vi "Setup.vi"(8 "error in":errorcluster, 11 "LUnit Test Commands In":refnum<class "Test Commands.lvclass">) -> (0 "error out":errorcluster, 3 "LUnit Test Commands Out":refnum<class "Test Commands.lvclass">)   [LabVIEW 2019, in "Test Commands.lvclass"]
doc: "Setup method called by the testing framework to set up test fixture before each test method is called."
uses:
  Test Commands.lvclass
  Test Commands.lvclass/Test Commands.ctl
  <vilib>/Astemes/LUnit/Test Case.lvclass
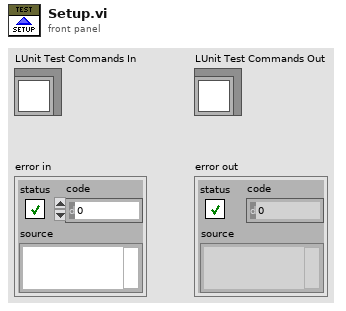
[diagram p1: front panel]
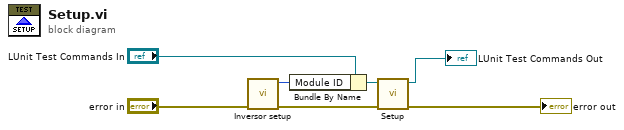
[diagram p0: block diagram]
diagram:
  n1 = call "Inversor setup.vi"("error in (no error)"="error in") -> ("error out"=w5:errorcluster, "Module ID"=w1:i32)  [unwired: 9 in]
  n2 = Bundle By Name(cluster="LUnit Test Commands In", "Module ID"=w1) -> (w2:refnum<class "Test Commands.lvclass">)
  n3 = call-parent "Setup.vi"("error in (no error)"=w5, "LUnit Test Case In"=w2) -> ("error out"=→"error out":errorcluster, "LUnit Test Case Out"=→"LUnit Test Commands Out":refnum<class "Test Commands.lvclass">)  [unwired: 8 in]
